vi "EndOfPathHandler.vi"(8 "MaxAccel":dbl, 9 "MaxVel":dbl, 10 "RobotLocation":cluster{dbl, dbl}, 11 "Path":cluster{"x":dbl, "y":dbl}[](array[cluster])=[{"x"=0.0, "y"=10.0}, {"x"=0.0, "y"=80.0}, {"x"=85.0, "y"=140.0}, {"x"=85.0, "y"=20.0}, {"x"=40.0, "y"=15.0}]) -> (0 "Done":bool, 1 "Override":bool, 2 "ExtraPowerOut":dbl, 3 "VelOut":dbl)   [LabVIEW 2016]
uses:
  <vilib>/addons/control/pid/pid.llb/PID (DBL).vi
  <vilib>/addons/control/pid/NI_PID_pid.lvlib
panel:
  in  "PID gains":T1 {"derivative time (Td, min)" format="%.3f"; "integral time (Ti, min)" format="%.3f"; "proportional gain (Kc)" format="%.3f"}
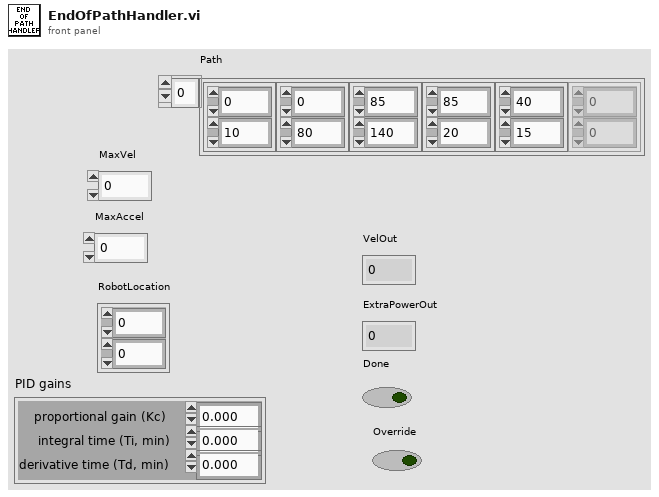
[diagram p1: front panel]
types:
  T1 = cluster{"proportional gain (Kc)":dbl, "integral time (Ti, min)":dbl, "derivative time (Td, min)":dbl}
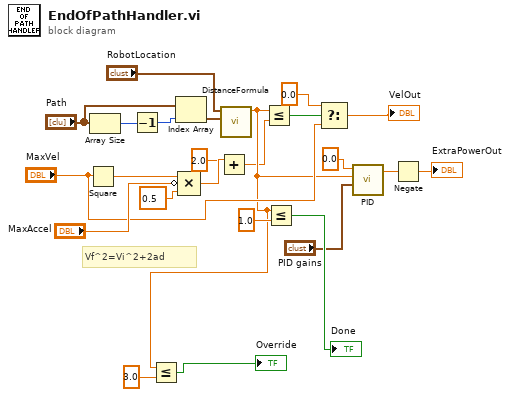
[diagram p0: block diagram]
diagram:
  # "Vf^2=Vi^2+2ad"
  n1 = Square(x="MaxVel") -> (x^2=w24:dbl)
  n2 = Array Size(array="Path") -> (size(s)=w21:i32)
  n3 = Decrement(x=w21) -> (x-1=w20:i32)
  n4 = Index Array(array="Path", index=w20) -> (element=w18:cluster{"x":dbl, "y":dbl})
  n5 = Compound Arithmetic op=MULTIPLY(w24, invert "MaxAccel", 0.5 ("value")) -> (w3:dbl)
  n6 = Add(x=w3, y=2.0) -> (x+y=w1:dbl)
  n7 = call "DistanceFormula.vi"("Point 2"=w18, "Point 1"="RobotLocation") -> ("Distance"=w5:dbl)  [unwired: 9 in]
  n8 = Less Or Equal?(x=w5, y=3.0) -> (x <= y?=→"Override":bool)
  n9 = Less Or Equal?(x=w5, y=w1) -> (x <= y?=w14:bool)
  n10 = Less Or Equal?(x=w5, y=1.0) -> (x <= y?=→"Done":bool)
  n11 = Select(t=0.0, s=w14, f="MaxVel") -> (s? t:f=→"VelOut":dbl)
  n12 = call-poly <vilib>:"PID.vi"("PID gains"="PID gains", "process variable"=w5, "setpoint"=0.0) -> ("output"=w8:dbl)  [unwired: 7 in, 1 out]
  n13 = Negate(x=w8) -> (-x=→"ExtraPowerOut":dbl)
